vi "FTW-Regex-FilterArray.vi"(0 "Regex Filter":string, 5 "Input Array":string[](array[string]), 11 "error in":errorcluster) -> (6 "Matching Items":string[](array[string]), 8 "Regex Results":cluster{"Match":string, "Submatches":string[]}[](array[cluster]), 15 "error out":errorcluster)   [LabVIEW 2014]
uses:
  Error/FTW-ERR-ThrowError.vi
panel:
  # "Inputs"
  # "Outputs"
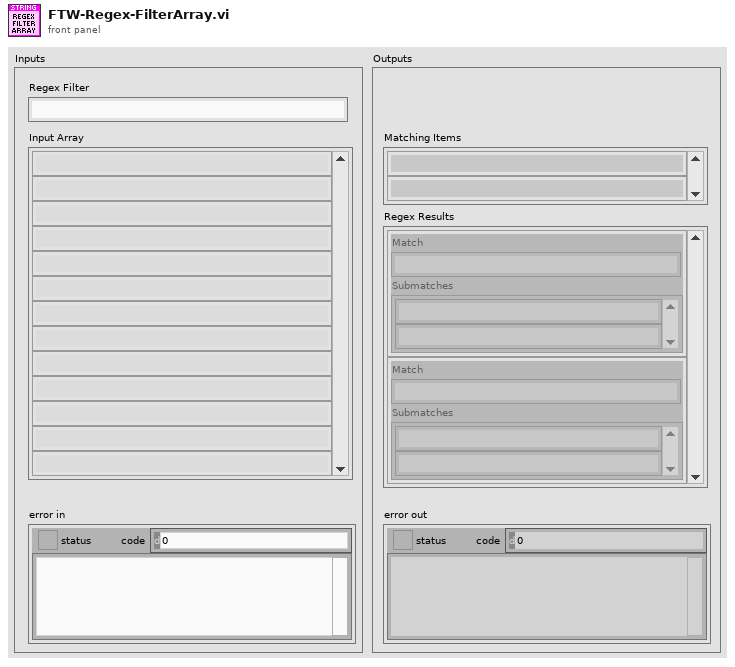
[diagram p1: front panel]
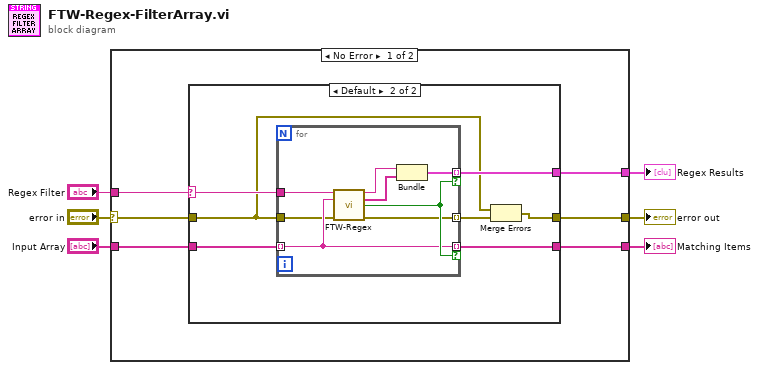
[diagram p0: block diagram]
diagram:
  n1 = case shown="No Error" "error in" {
    selector: "error in" -> [w7 w30]
    tunnel: [w9 w30] -> w6
    tunnel: "Regex Filter" -> [w12 _]
    tunnel: [w10 _] -> w3
    tunnel: [w11 _] -> w1
    tunnel: "Input Array" -> [w8 _]
    frame No Error {
      n2 = case shown="Default" w12 {
        selector: w12 -> [_ w20]
        tunnel: w8 -> [w14 w21]
        tunnel: [w14 w19] -> w10
        tunnel: [_ w18] -> w11
        tunnel: [w13 w16] -> w9
        tunnel: w7 -> [w13 w15]
        frame "" {
          # "Just return everything"
        }
        frame Default {
          n3 = for {
            tunnel: w21 -> [w25] mode=indexing
            tunnel: w20 -> [w26]
            tunnel: [w25] -> w19 mode=indexing if=w28
            tunnel: [w29] -> w18 mode=indexing if=w28
            tunnel: w15 -> [w24]
            tunnel: [w23] -> w17 mode=indexing
            n4 = call "FTW-Regex.vi"("Regular Expression"=w26, "Input String"=w25, "error in"=w24) -> ("Match"=w22:string, "Submatches"=w27:string[], "Match Found?"=w28:bool, "error out"=w23:errorcluster)  [unwired: 8 in, 1 out]
            n5 = Bundle("Match"=w22, "Submatches"=w27) -> (w29:cluster{"Match":string, "Submatches":string[]})  [unwired: 1 in]
          }
          n6 = Merge Errors(w15, w17) -> (w16:errorcluster)
        }
      }
    }
    frame Error {
    }
  }
  "error out" <- w6
  "Matching Items" <- w3
  "Regex Results" <- w1
